vi "STRAIN_MAIN.vi"() -> ()   [LabVIEW 2019]
uses:
  <vilib>/ptbypt/NI_PtbyPt.lvlib
panel:
  in  "退出":T1
  in  "串口读取":bool
  in  "选项卡控件":enum32{"采集配置", "图形显示", "雨流计数法", "数据保存"}(tab)
  in  "串口设置":T2={"波特率"=9600, "数据位"=8, "校验"=enum."None", "停止位"=10, "VISA资源名称"="COM1", "XON"=enum."DC1", "XOFF"=enum."DC3", "终止符时结束读取？"=TRUE, "终止符"=10, "流控制"=0} {"流控制" items=["无"=0, "XON/XOFF"=1, "RTS/CTS"=2, "DTR/DSR"=4]; "终止符" format="%.0x"; "停止位" items=["1.0"=10, "1.5"=15, "2.0"=20]; "数据位" min=5 max=8 step=1; "波特率" items=["75"=75, "110"=110, "134"=134, "150"=150, "300"=300, "600"=600, "1200"=1200, "1800"=1800, "2400"=2400, "4800"=4800, "7200"=7200, "9600"=9600, "14400"=14400, "19200"=19200, "28800"=28800, "38400"=38400, "56000"=56000, "57600"=57600, "115200"=115200, "128000"=128000, "230400"=230400]}
  out "数据接收":string
  in  "数据发送":cluster{"命令":string, "是否写入":bool}={"命令"="*IDN?", "是否写入"=FALSE}
  out "波形图表 2":dbl(graph)
  out "波形图表":dbl(graph)
  in  "应变数据转换配置":T3={"电桥"="全桥", "ADC精度"=24.0, "增益倍数"=128.0, "参考电压"=4.3, "应变片灵敏度"=2.2}
  out "Cluster 2":T4
  out "Cluster":T5
  in  "?":bool
  out "数组 - 字符串":string[][](array[string])
  in  "数据筛选":cluster{"实验ID筛选":string, "应变值筛选":string}
  in  "数据库配置":T6
  # "1280*800"
  # "1.一律使用“银色”风格控件\n2.一律使用自带控件，非必要，不自定义控件\n3.\n4.\n5.\n6."
  # "船   舶   健   康   监   测   系   统"
  # "串口通讯"
  # "电桥配置"
  # "数据链接："
  # "实验标签："
  # "列名3："
  # "列名2："
  # "列名1："
  # "写入表名："
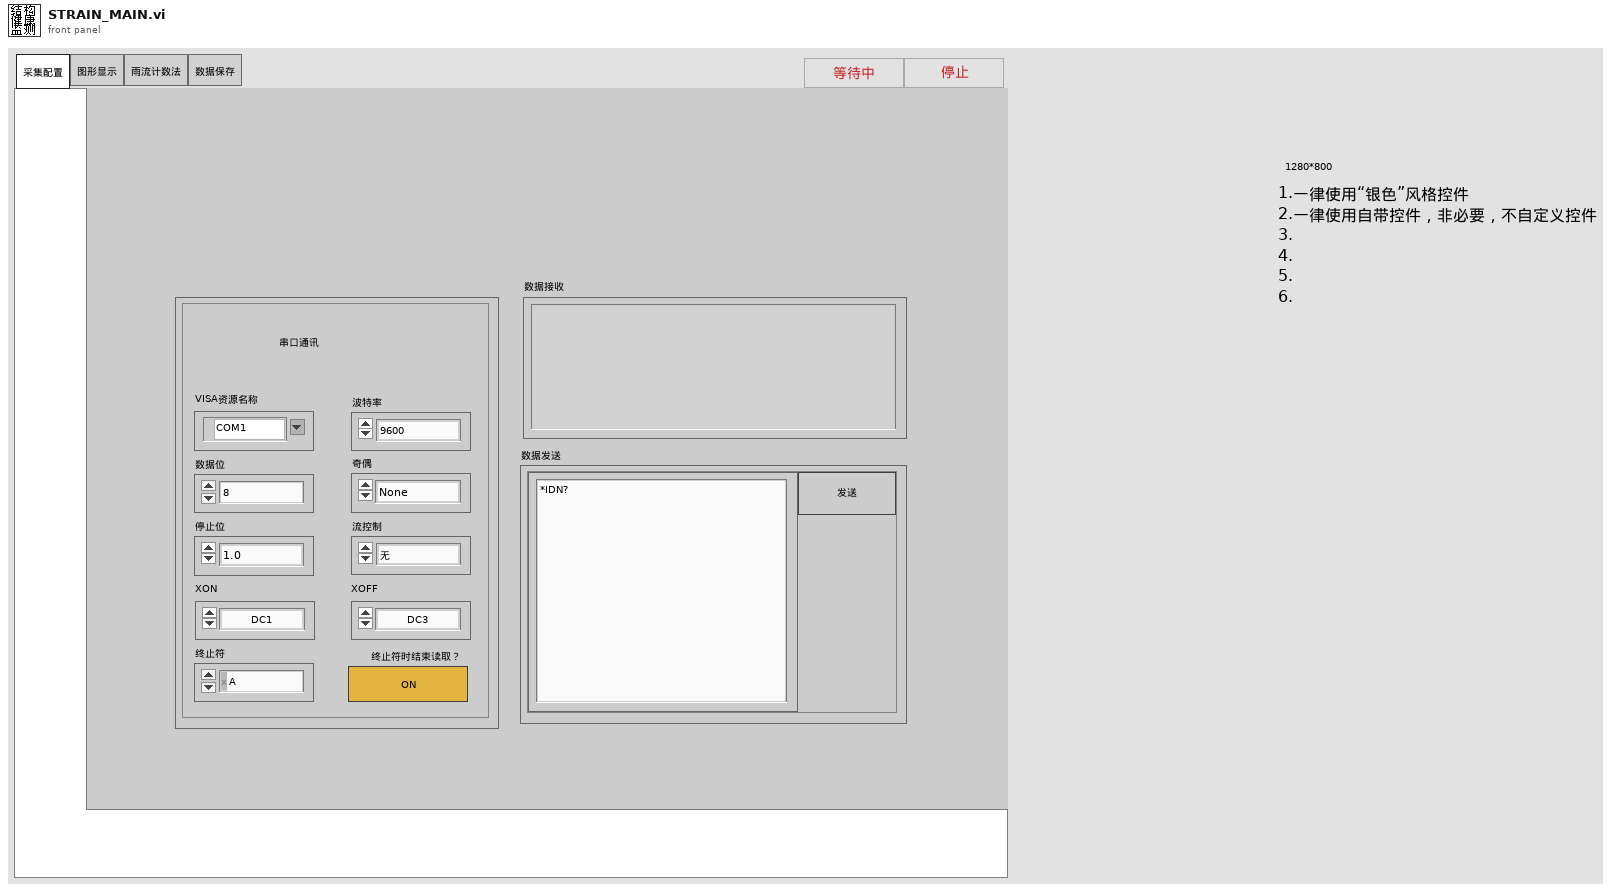
[diagram p1: front panel]
types:
  T1 = typedef "控件 1.ctl" = bool
  T2 = cluster{"波特率":u32, "数据位":u16, "校验":enum16{"None", "Odd", "Even", "Mark", "Space"}, "停止位":u16, "VISA资源名称":refnum<visa-resource-name>, "XON":enum16{"NUL", "SOH", "STX", "ETX", "EOT", "ENQ", "ACK", "BEL", "BS", "HT", "LF", "VT", "FF", "CR", "SO", "SI", "DLE", "DC1", "DC2", "DC3", "DC4", "NAK", "SYN", "ETB", "CAN", "EM", "SUB", "ESC", "FS", "GS", "RS", "US", "SP", "!", "\"", "#", "$", "%", "&", "'", "(", ")", "*", "+", ",", "- (-)", ".", "/", "0", "1", "2", "3", "4", "5", "6", "7", "8", "9", ":", ";", "<", "=", ">", "?", "@", "A", "B", "C", "D", "E", "F", "G", "H", "I", "J", "K", "L", "M", "N", "O", "P", "Q", "R", "S", "T", "U", "V", "W", "X", "Y", "Z", "[", "\\", "]", "^", "_", "`", "a", "b", "c", "d", "e", "f", "g", "h", "i", "j", "k", "l", "m", "n", "o", "p", "q", "r", "s", "t", "u", "v", "w", "x", "y", "z", "{", "|", "}", "~"}, "XOFF":enum16{"NUL", "SOH", "STX", "ETX", "EOT", "ENQ", "ACK", "BEL", "BS", "HT", "LF", "VT", "FF", "CR", "SO", "SI", "DLE", "DC1", "DC2", "DC3", "DC4", "NAK", "SYN", "ETB", "CAN", "EM", "SUB", "ESC", "FS", "GS", "RS", "US", "SP", "!", "\"", "#", "$", "%", "&", "'", "(", ")", "*", "+", ",", "- (-)", ".", "/", "0", "1", "2", "3", "4", "5", "6", "7", "8", "9", ":", ";", "<", "=", ">", "?", "@", "A", "B", "C", "D", "E", "F", "G", "H", "I", "J", "K", "L", "M", "N", "O", "P", "Q", "R", "S", "T", "U", "V", "W", "X", "Y", "Z", "[", "\\", "]", "^", "_", "`", "a", "b", "c", "d", "e", "f", "g", "h", "i", "j", "k", "l", "m", "n", "o", "p", "q", "r", "s", "t", "u", "v", "w", "x", "y", "z", "{", "|", "}", "~"}, "终止符时结束读取？":bool, "终止符":u8, "流控制":u16}
  T3 = cluster{"电桥":string, "ADC精度":dbl, "增益倍数":dbl, "参考电压":dbl, "应变片灵敏度":dbl}
  T4 = cluster{"4.均值":cluster{"子数组2":i32[], "子数组1":dbl[]}, "5.幅值":cluster{"子数组2":i32[], "子数组1":dbl[]}}
  T5 = cluster{"1.载荷源数据":cluster{"Data":i32[], "label":i32[]}, "2.提取波峰波谷数据":cluster{"时间戳":i32[], "峰谷戳":i32[]}, "3.载荷历程数据":cluster{"子数组1":i32[], "子数组2":i32[]}}
  T6 = cluster{"String":string, "String 2":string, "String 3":string, "String 4":string, "String 5":string, "String 6":string}
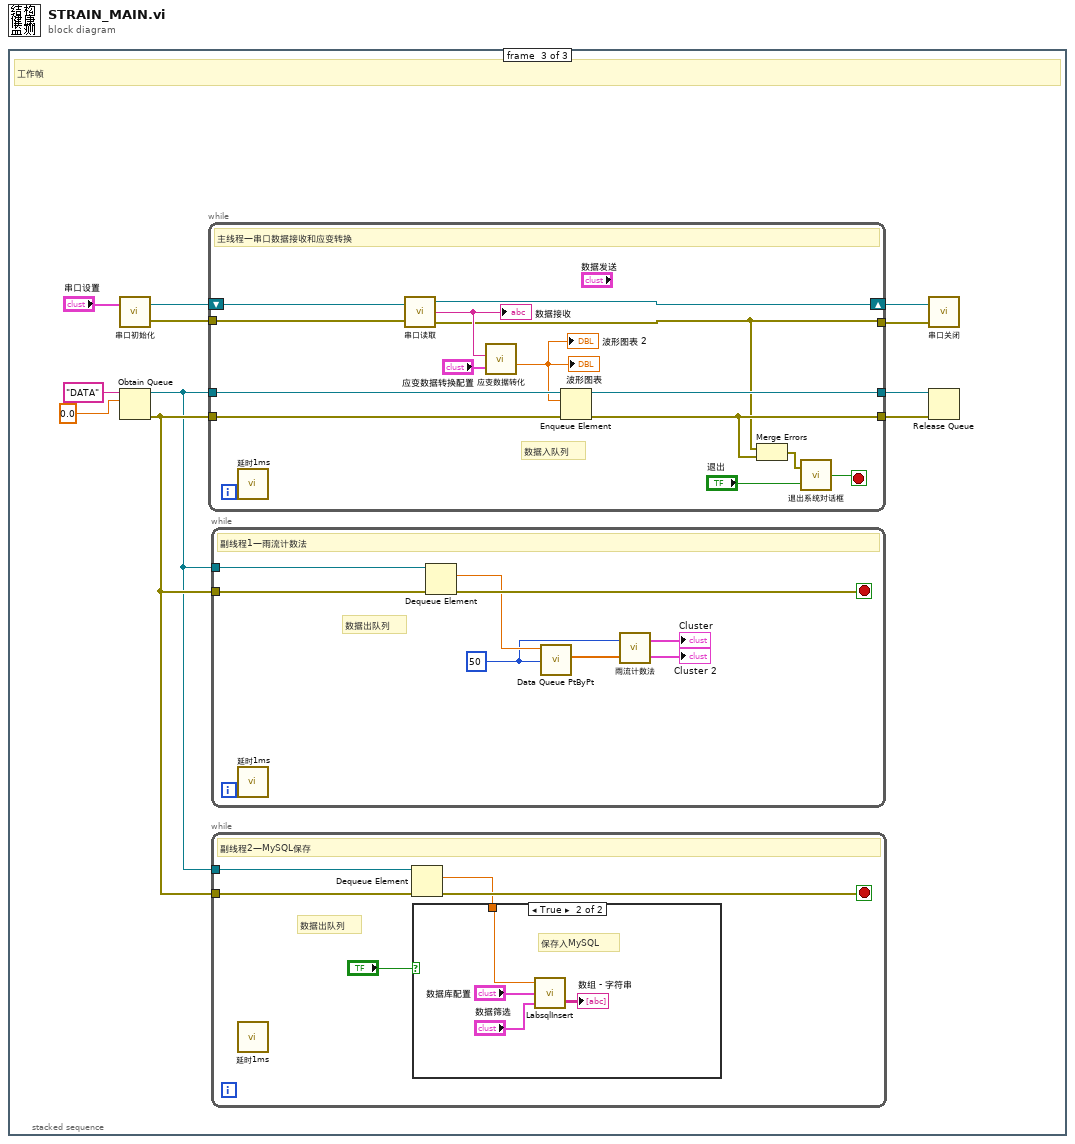
[diagram p0: block diagram]
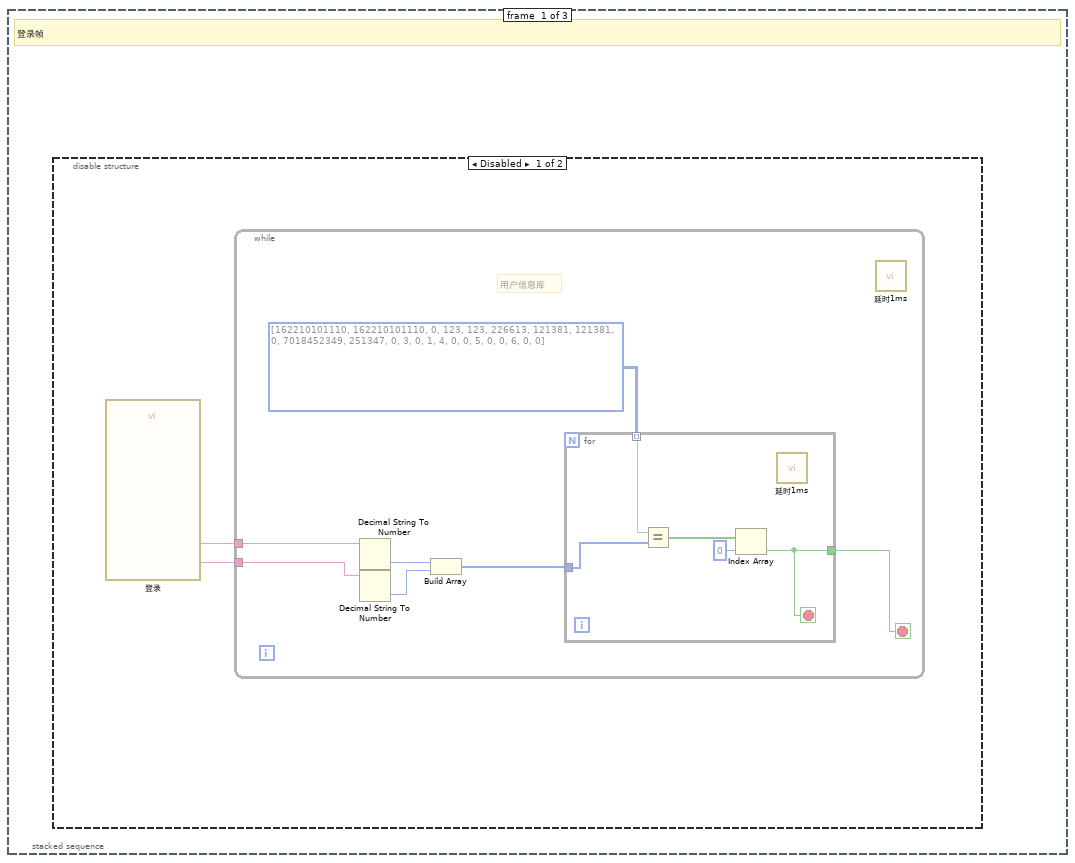
[diagram p2: hidden frame]
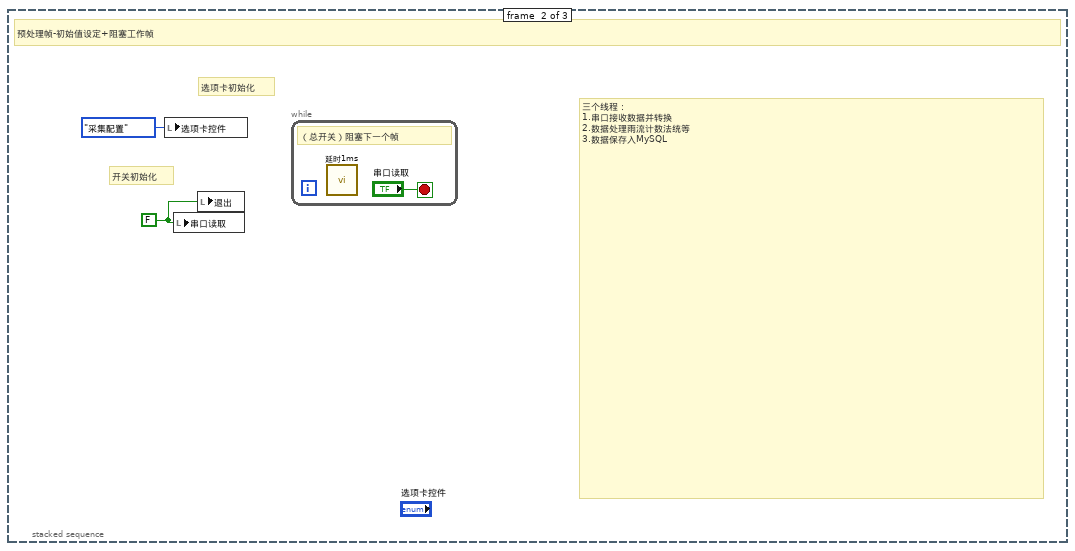
[diagram p4: hidden frame]
diagram:
  n1 = stacked-sequence {
    frame #0 {
      # "登录帧"
      n2 = disable-structure shown="Disabled" {
        frame Disabled {
          n3 = call "登录"() -> ("密码"=w2:string, "用户名"=w1:string)  [unwired: 16 in, 2 out]
          n4 = while {
            tunnel: w2 -> [w5]
            tunnel: w1 -> [w4]
            stop <- w3 stop-if-true
            # "用户信息库"
            n5 = Decimal String To Number(string=w4) -> (number=w8:i32)  [unwired: 2 in, 1 out]
            n6 = Decimal String To Number(string=w5) -> (number=w7:i32)  [unwired: 2 in, 1 out]
            n7 = Build Array(w8, w7) -> (w6:i32[])
            n8 = for {
              tunnel: u64[][] [[162210101110, 162210101110, 0], [123, 123, 226613], [121381, 121381, 0], [7018452349, 251347, 0], [3, 0, 1], [4, 0, 0], [5, 0, 0], [6, 0, 0]] -> [w14] mode=indexing
              tunnel: w6 -> [w10]
              tunnel: [w11] -> w3
              stop <- w11 stop-if-true
              n9 = Equal?(x=w14, y=w10) -> (x = y?=w13:bool[])
              n10 = Index Array(array=w13, index=0 ("索引")) -> (element=w11:bool)
              n11 = call "延时1ms.vi"() -> ()  [unwired: 12 in]
            }
            n12 = call "延时1ms.vi"() -> ()  [unwired: 12 in]
          }
        }
        frame Enabled {
        }
      }
    }
    frame #1 {
      w16 = FALSE ("保存数据")
      # "三个线程：\n1.串口接收数据并转换\n2.数据处理雨流计数法统等\n3.数据保存入MySQL"
      # "选项卡初始化"
      # "开关初始化"
      # "预处理帧-初始值设定+阻塞工作帧"
      n13 = local write "选项卡控件"(enum32{"采集配置", "图形显示", "雨流计数法", "数据保存"}."采集配置" ("选项卡控件")) -> ()
      n14 = local write "串口读取"(w16) -> ()
      n15 = local write "退出"(w16) -> ()
      n16 = while {
        stop <- "串口读取" stop-if-true
        # "（总开关）阻塞下一个帧"
        n17 = call "延时1ms.vi"() -> ()  [unwired: 12 in]
      }
    }
    frame #2 {
      # "工作帧"
      n18 = call "串口初始化.vi"("串口设置"="串口设置") -> ("错误输出"=w23:errorcluster, "VISA resource name out"=w21:refnum<visa-resource-name>)  [unwired: 1 in]
      n19 = Obtain Queue(name (unnamed)="DATA" ("名称（未命名）"), element data type=0.0 ("波形图表")) -> (queue out=w27:refnum<queue>, error out=w28:errorcluster)  [unwired: 3 in, 1 out]
      n20 = while {
        shift-right: [w47] -> w20
        shift-left: w21 -> [w59]
        tunnel: w23 -> [w58]
        tunnel: [w46] -> w24
        tunnel: w27 -> [w55]
        tunnel: w28 -> [w54]
        tunnel: [w53] -> w25
        tunnel: [w52] -> w26
        stop <- w56 stop-if-true
        # "数据入队列"
        # "主线程—串口数据接收和应变转换"
        n21 = call "延时1ms.vi"() -> ()  [unwired: 12 in]
        n22 = call "串口读取.vi"("VISA resource name in"=w59, "错误输入（无错误）"=w58) -> ("VISA resource name out"=w47:refnum<visa-resource-name>, "响应"=w50:string, "错误输出"=w46:errorcluster)
        "数据接收" <- w50
        n23 = call "应变数据转化.vi"("应变数据转换配置"="应变数据转换配置", "原始数据入"=w50) -> ("应变"=w48:dbl)
        "波形图表" <- w48
        "波形图表 2" <- w48
        n24 = Enqueue Element(queue=w55, element=w48, error in (no error)=w54) -> (queue out=w53:refnum<queue>, error out=w52:errorcluster)  [unwired: 1 in, 1 out]
        n25 = Merge Errors(w46, w52) -> (w51:errorcluster)
        n26 = call "退出系统对话框.vi"("退出"="退出", "error in (no error)"=w51) -> ("T/F"=w56:bool)
      }
      n27 = while {
        tunnel: w27 -> [w45]
        tunnel: w28 -> [w44]
        stop <- w43 stop-if-true
        w38 = 50 ("sample length")
        # "数据出队列"
        # "副线程1—雨流计数法"
        n28 = call "延时1ms.vi"() -> ()  [unwired: 12 in]
        n29 = Dequeue Element(queue=w45, error in (no error)=w44) -> (element=w42:dbl, error out=w43:errorcluster)  [unwired: 1 in, 2 out]
        n30 = call <vilib>:"Data Queue PtByPt.vi"("sample length"=w38, "input data point"=w42) -> ("Current Queue"=w41:dbl[])  [unwired: 5 in, 4 out]
        n31 = call "雨流计数法.vi"("Data"=w41, "数据个数"=w38) -> ("Cluster 2"=→"Cluster 2":T4, "Cluster"=→"Cluster":T5)
      }
      n32 = while {
        tunnel: w27 -> [w33]
        tunnel: w28 -> [w32]
        stop <- w31 stop-if-true
        # "数据出队列"
        # "副线程2—MySQL保存"
        n33 = call "延时1ms.vi"() -> ()  [unwired: 12 in]
        n34 = Dequeue Element(queue=w33, error in (no error)=w32) -> (element=w30:dbl, error out=w31:errorcluster)  [unwired: 1 in, 2 out]
        n35 = case shown="True" "?" {
          tunnel: w30 -> [_ w37]
          frame False {
          }
          frame True {
            # "保存入MySQL"
            n36 = call "LabsqlInsert.vi"("Cluster"="数据筛选", "数据库配置"="数据库配置", "存入的应变值"=w37) -> ("数组 - 字符串"=→"数组 - 字符串":string[][])  [unwired: 1 out]
          }
        }
      }
      n37 = call "串口关闭.vi"("错误输入（无错误）"=w24, "VISA资源名称"=w20) -> ()  [unwired: 1 in]
      n38 = Release Queue(queue=w25, error in (no error)=w26) -> ()  [unwired: 1 in, 3 out]
    }
  }
